vi "rising edge rate counter.vi"(9 "threshold":sgl=0.5, 10 "sample_rate":sgl, 11 "Data Array":sgl[](array[numeric])) -> (3 "Array out":sgl[](array[numeric]))   [LabVIEW 2021, in "libad4.lvlib"]
doc: "Software based rising edge period."
uses:
  <userlib>/libad4/libad4.lvlib
  7bcf6d59-b17f-4243-b144-ab4d2688ffc3.vi
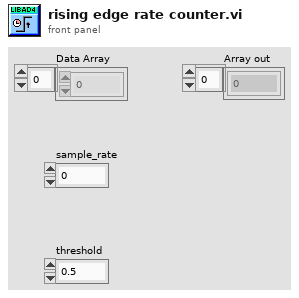
[diagram p1: front panel]
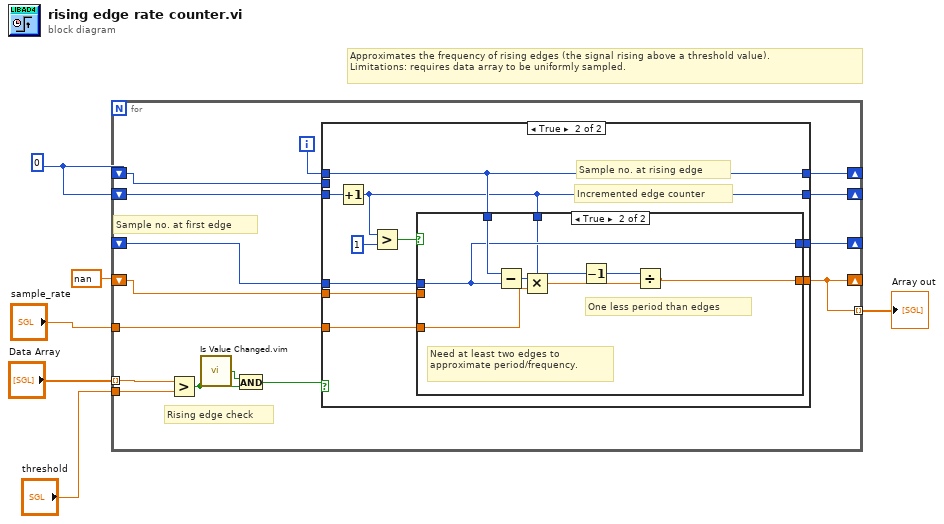
[diagram p0: block diagram]
diagram:
  w2 = 0
  # "Approximates the frequency of rising edges (the signal rising above a threshold value). \nLimitations: requires data array to be uniformly sampled."
  n1 = for {
    tunnel: "Data Array" -> [w20] mode=indexing
    shift-right: [w16] -> _
    shift-left: w2 -> [w7]
    tunnel: "sample_rate" -> [w12]
    tunnel: "threshold" -> [w21]
    shift-right: [w13] -> _
    shift-left: w2 -> [w14]
    shift-right: [w9] -> _
    shift-left: nan -> [w8]
    tunnel: [w9] -> w3 mode=indexing
    shift-right: [w11] -> _
    shift-left: _ -> [w10]
    i -> [w15]
    # "Rising edge check"
    # "Sample no. at first edge"
    n2 = Greater?(x=w20, y=w21) -> (0:w18:bool)
    n3 = call "Is Value Changed.vim"("value"=w18) -> ("changed or first call?"=w19:bool)
    n4 = And(x=w19, y=w18) -> (x .and. y?=w17:bool)
    n5 = case shown="True" w17 {
      tunnel: w15 -> [_ w32]
      tunnel: [w23 w32] -> w16
      tunnel: w14 -> [w24 w35]
      tunnel: [w24 w28] -> w13
      tunnel: w12 -> [_ w31]
      tunnel: [w22 w30] -> w11
      tunnel: w10 -> [w22 w29]
      tunnel: [w25 w27] -> w9
      tunnel: w8 -> [w25 w26]
      tunnel: w7 -> [w23 _]
      frame False {
      }
      frame True {
        # "Incremented edge counter"
        # "Sample no. at rising edge"
        n6 = Increment(x=w35) -> (x+1=w28:i32)
        n7 = Greater?(x=w28, y=1) -> (0:w33:bool)
        n8 = case shown="True" w33 {
          tunnel: w32 -> [w37 w45]
          tunnel: w31 -> [_ w43]
          tunnel: [w37 w41] -> w30
          tunnel: w29 -> [_ w41]
          tunnel: w28 -> [_ w39]
          tunnel: [w36 w38] -> w27
          tunnel: w26 -> [w36 _]
          frame False {
          }
          frame True {
            # "One less period than edges"
            # "Need at least two edges to \napproximate period/frequency."
            n9 = Subtract(x=w45, y=w41) -> (x-y=w44:i32)
            n10 = Multiply(x=w44, y=w43) -> (x*y=w42:sgl)
            n11 = Decrement(x=w39) -> (x-1=w40:i32)
            n12 = Divide(x=w40, y=w42) -> (x/y=w38:sgl)
          }
        }
      }
    }
  }
  "Array out" <- w3
